vi "CTRE_Phoenix_CANdle_GetFirmwareVersion.vi"(8 "error in":errorcluster, 11 "CTRE_CANdle_DeviceRef":T1) -> (0 "error out":errorcluster, 2 "firmware version":i32, 3 "CTRE_CANdle_DeviceRef":T1)   [LabVIEW 2020]
doc: "Returns the device firmware version."
uses:
  <vilib>/Rock Robotics/WPI/ThirdParty/Phoenix-LabVIEW/CANdle/Controls/CTRE_Phoenix_CANdle_DeviceRef.ctl
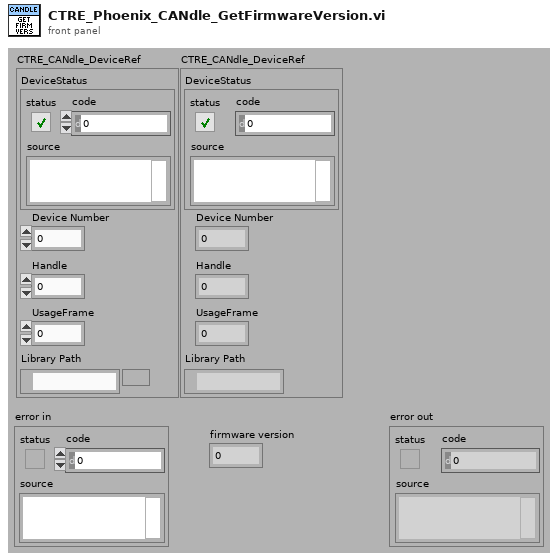
[diagram p1: front panel]
types:
  T1 = typedef "CTRE_Phoenix_CANdle_DeviceRef.ctl" = cluster{"DeviceStatus":errorcluster, "Device Number":u8, "Handle":u64, "UsageFrame":u32, "Library Path":path}
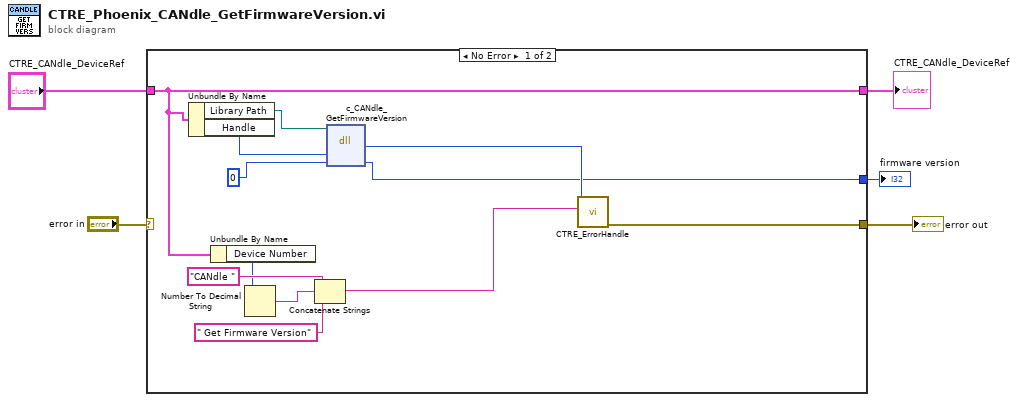
[diagram p0: block diagram]
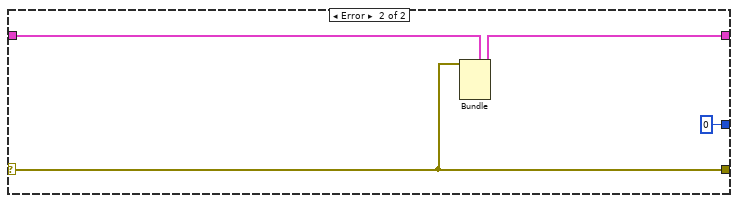
[diagram p2: hidden frame]
diagram:
  n1 = case shown="No Error" "error in" {
    selector: "error in" -> [_ w20]
    tunnel: "CTRE_CANdle_DeviceRef" -> [w8 w21]
    tunnel: [w16 w20] -> w5
    tunnel: [w8 w19] -> w1
    tunnel: [w9 0 ("percentOutput")] -> w3
    frame No Error {
      n2 = Unbundle By Name(w8) -> ("Library Path"=w7:path, "Handle"=w6:u64)
      n3 = Unbundle By Name(w8) -> ("Device Number"=w12:u8)
      n4 = Number To Decimal String(number=w12) -> (decimal integer string=w14:string)  [unwired: 1 in]
      n5 = Concatenate Strings("CANdle " ("string"), w14, " Get Firmware Version" ("string")) -> (w10:string)
      n6 = dll-call lib="?" fn="c_CANdle_GetFirmwareVersion"(path in=w7, "handle"=w6, "firmware"=u32 0 ("appliedThrottle")) -> ("return type"=w11:i32, "firmware"=w9:i32)  [unwired: 3 in, 2 out]
      n7 = call <vilib>:"CTRE_ErrorHandle.vi"("origin"=w10, "code"=w11) -> ("error out"=w16:errorcluster)  [unwired: 9 in]
    }
    frame Error {
      n8 = Bundle(cluster=w21, "DeviceStatus"=w20) -> (w19:T1)  [unwired: 4 in]
    }
  }
  "error out" <- w5
  "firmware version" <- w3
  "CTRE_CANdle_DeviceRef" <- w1
